vi "Process.vi"(8 "error in":errorcluster, 11 "instrument.Cryostation":refnum<class "instrument.Cryostation.lvclass">) -> (0 "error out":errorcluster, 3 "instrument.Cryostation out":refnum<class "instrument.Cryostation.lvclass">)   [LabVIEW 2019, in "instrument.Cryostation.lvclass"]
doc: "---------------------------------------------------------------\nJKI State Machine Objects™\nhttp://jki.net/state-machine-objects/\nCopyright (C) 2005-2015, JKI <info@jki.net>\nALL RIGHTS RESERVED"
uses:
  instrument.Cryostation.lvclass
  <vilib>/JKI/JKI SMO/SMO/SMO.lvclass
  C:/Program Files/National Instruments/LabVIEW 2019/user.lib/LevyLab/Instrument Framework/Instrument Types/Cryostat/Instrument.Cryostat.lvclass
  C:/Program Files/National Instruments/LabVIEW 2019/user.lib/LevyLab/Instrument Framework/Instrument/Instrument.lvclass
  C:/Program Files/National Instruments/LabVIEW 2019/vi.lib/JKI/JKI SMO/SMO/SMO.lvclass
  <userlib>/LevyLab/Debug/Debug.lvlib
  <userlib>/LevyLab/Instrument Framework/Instrument/Instrument.lvclass
  <userlib>/LevyLab/Instrument Framework/Instrument Types/Cryostat/Instrument.Cryostat.lvclass
panel:
  out "status string":string
  out "State History":string
  in  "STOP":bool
  # "Montana Cryostation"
  # "Montana Cryostation Monitor"
  # "THIS ONE IS NOT THE UI"
  # "For instructions on how to use the JKI State Machine Objects, examples and video tutorials, visit:\nhttp://jki.net/state-machine-objects/\n\nJKI State Machine Objects™\nhttp://jki.net/state-machine-objects/\nCopyright (C) 2005-2015, JKI <info@jki.net>\nALL RIGHTS RESERVED"
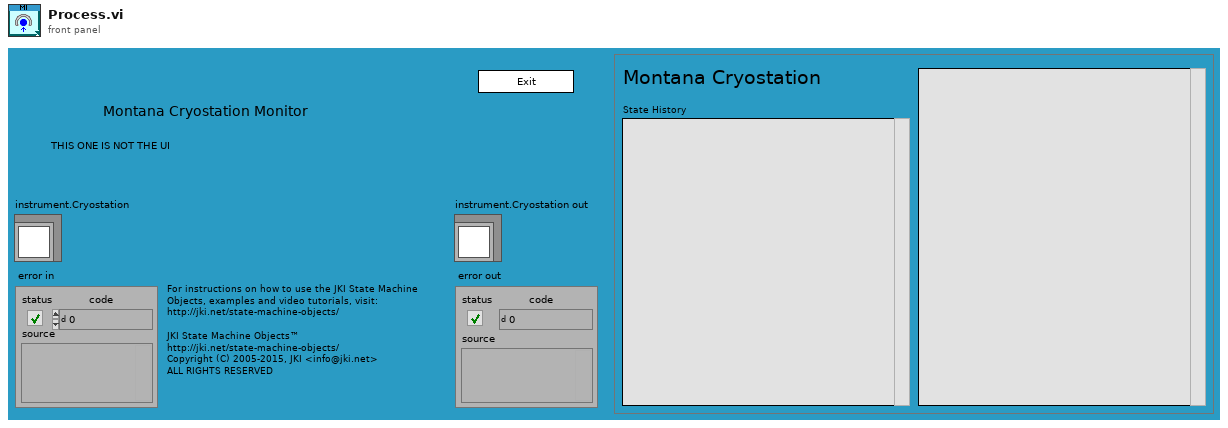
[diagram p1: front panel]
types:
  T1 = enum32{"invalid app kind", "Development System", "Run Time System", "Student Edition", "Embedded LabVIEW", "Evaluation", "Custom"}
  T2 = enum32{"Invalid", "Standard", "Closed", "Hidden", "Minimized", "Maximized"}
  T3 = cluster{"Core":cluster{"Current VI Reference":refnum<vi>, "Close Panel on Exit?":bool, "Shutdown?":bool, "Last Error":cluster{"error":errorcluster, "previous state":string, "remaining states":string}}, "SMO":refnum<class "instrument.Cryostation.lvclass">}
  T4 = cluster{"Current VI Reference":refnum<vi>, "Close Panel on Exit?":bool, "Shutdown?":bool, "Last Error":cluster{"error":errorcluster, "previous state":string, "remaining states":string}}
  T5 = typedef "Debug.lvlib/Attribute.Debug.lvclass/DebugBehavior.ctl" = enum16{"Normal", "Debug"}
  T6 = typedef "SMO.lvclass/Protected Events.ctl" = cluster{"StopProcesses":refnum<user-event>, "AbortProcesses":refnum<user-event>, "Config Changed":refnum<user-event>, "Dependency":refnum<user-event>}
  T7 = typedef "instrument.Cryostation.lvclass/Cryostation.getAll--cluster.ctl" = cluster{"Chamber Pressure (mTorr)":dbl, "Compressor Return Pressure (MPa)":dbl, "Compressor Supply Pressure (MPa)":dbl, "Compressor Speed (Hz)":dbl, "Cold Head Speed (Hz)":dbl, "Platform Heater Power (W)":dbl, "Platform Stability (K)":dbl, "Platform Temperature (K)":dbl, "Stage 1 Heater Power (W)":dbl, "Stage 1 Temperature (K)":dbl, "Stage 2 Heater Power (W)":dbl, "Stage 2 Temperature (K)":dbl, "Sample Stability (K)":dbl, "Sample Temperature (K)":dbl, "Temperature Set Point (K)":dbl, "User Stability (K)":dbl, "User Temperature (K)":dbl, "User Temperature Set Point (K)":dbl, "Alarm State":string, "Compressor Run State":string, "Case Valve State":string, "Idle State":string, "Nitrogen State":string, "Vent Valve State":string}
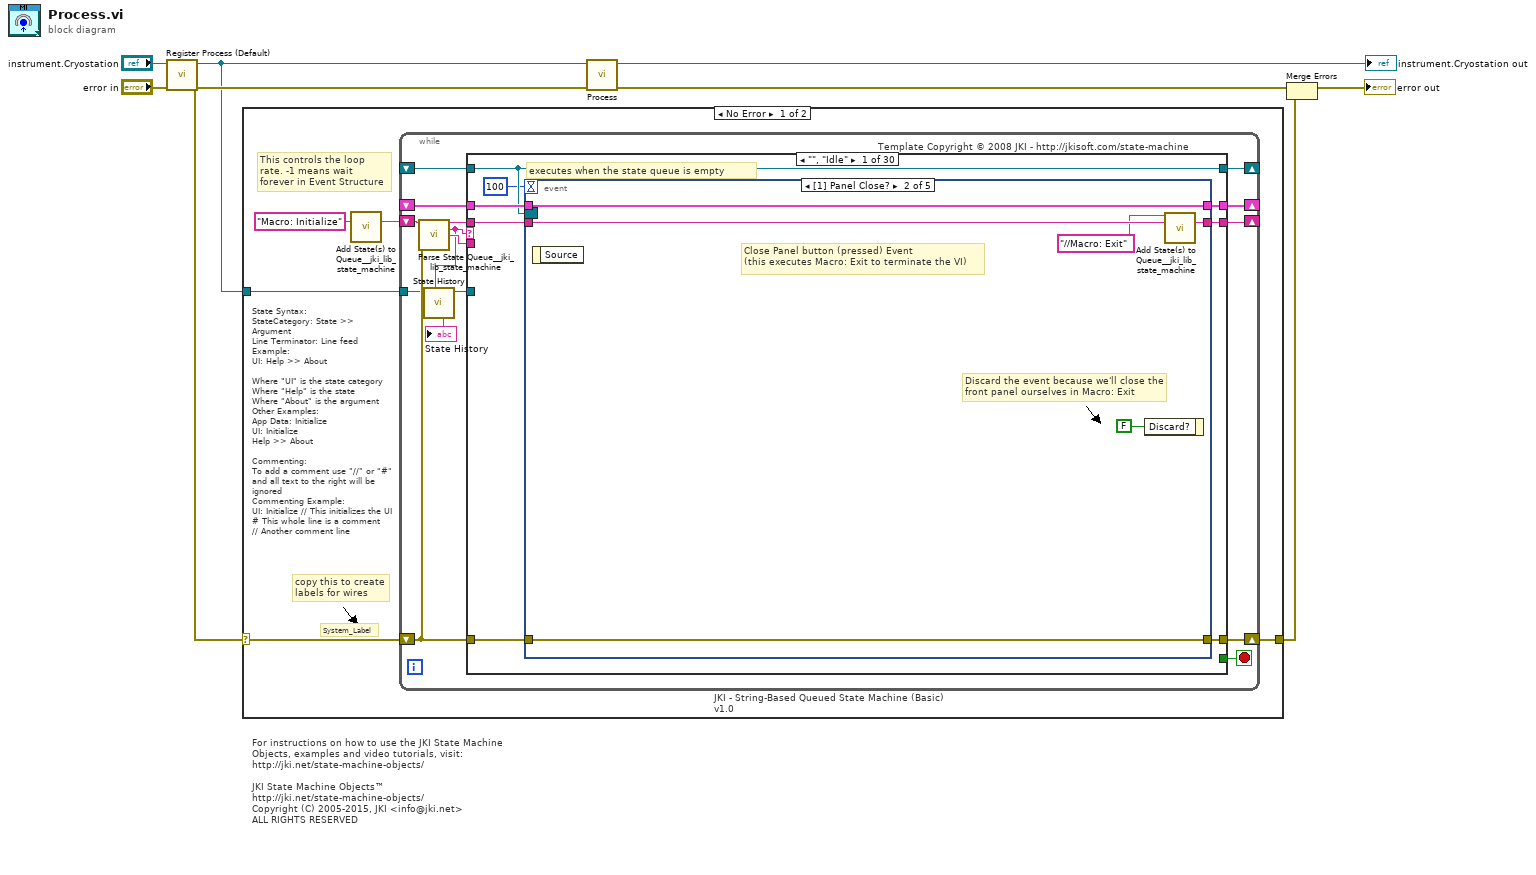
[diagram p0: block diagram]
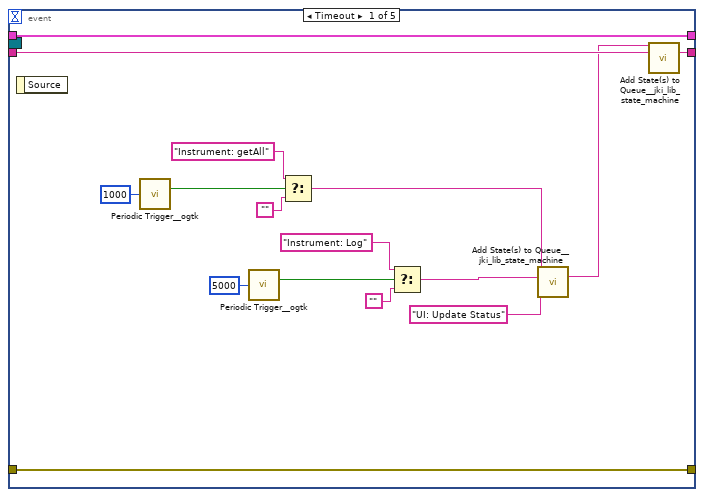
[diagram p2: hidden frame]
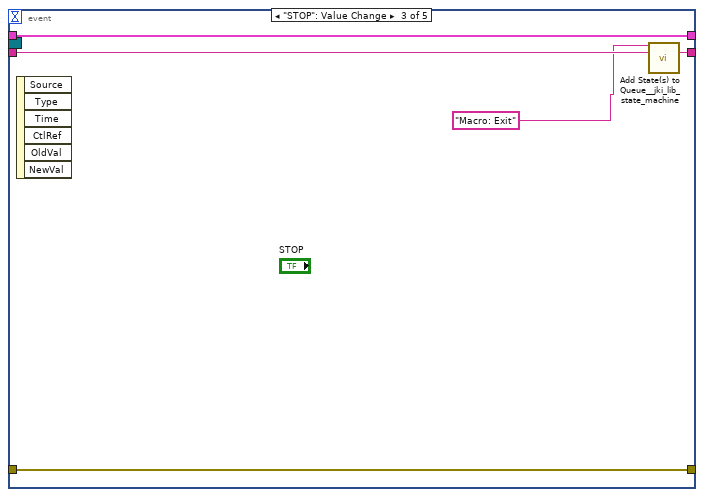
[diagram p3: hidden frame]
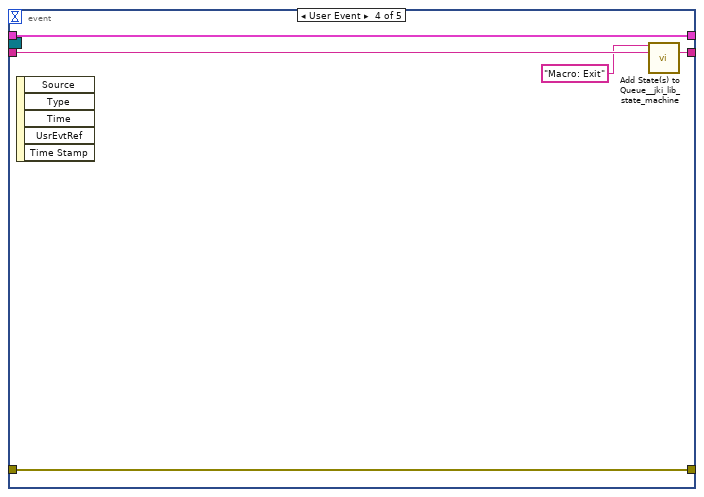
[diagram p4: hidden frame]
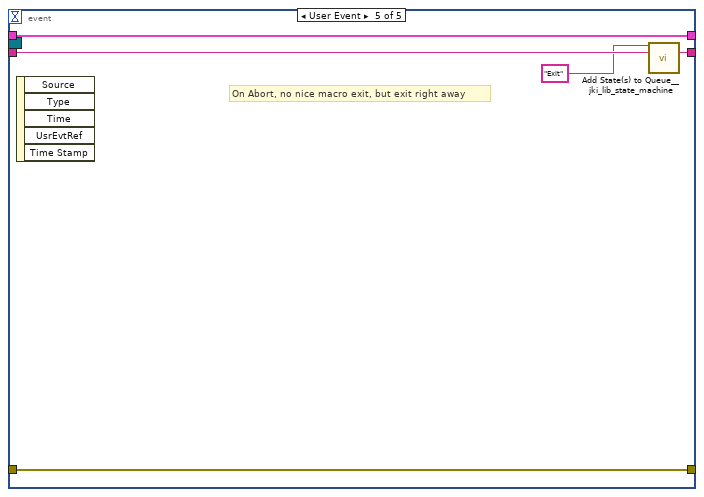
[diagram p5: hidden frame]
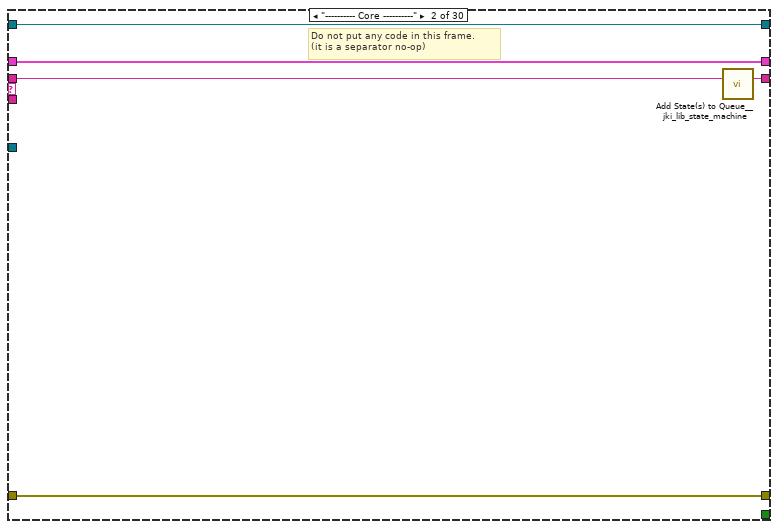
[diagram p6: hidden frame]
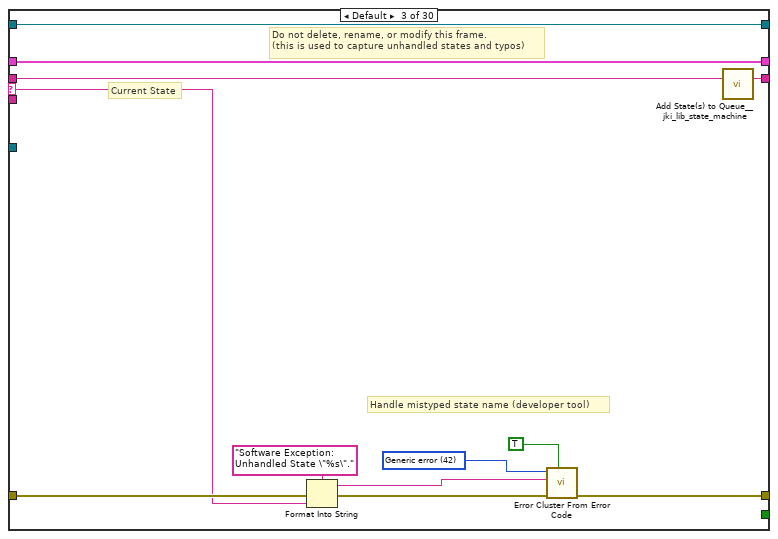
[diagram p7: hidden frame]
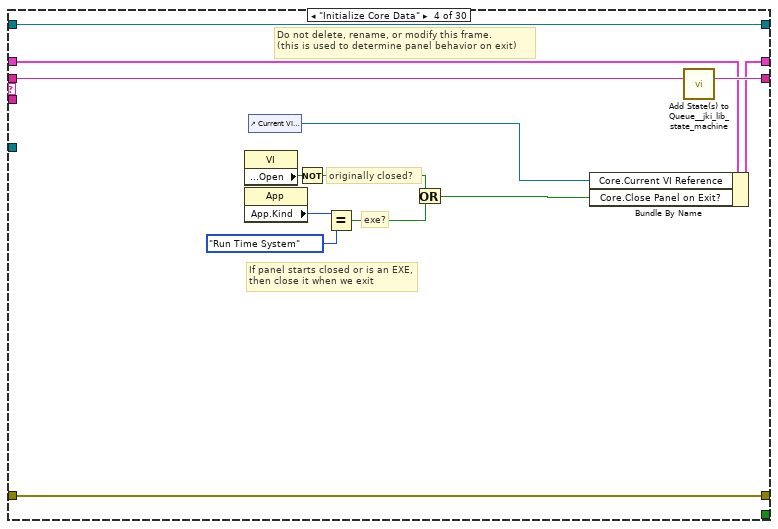
[diagram p8: hidden frame]
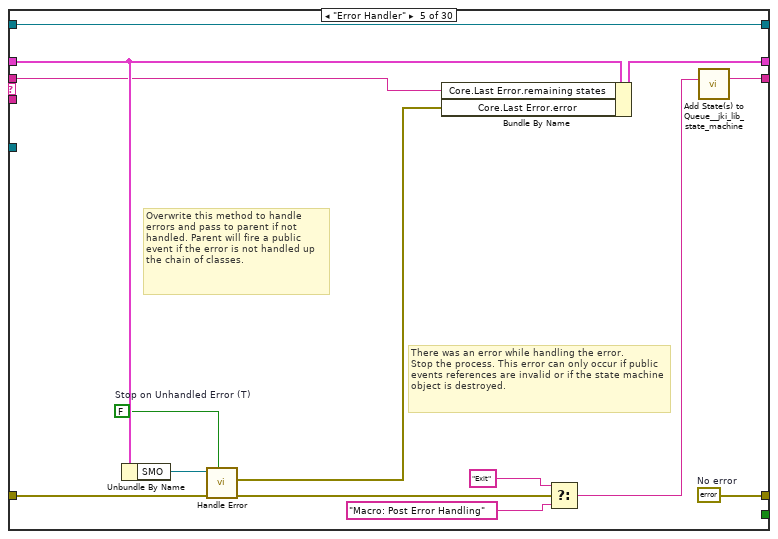
[diagram p9: hidden frame]
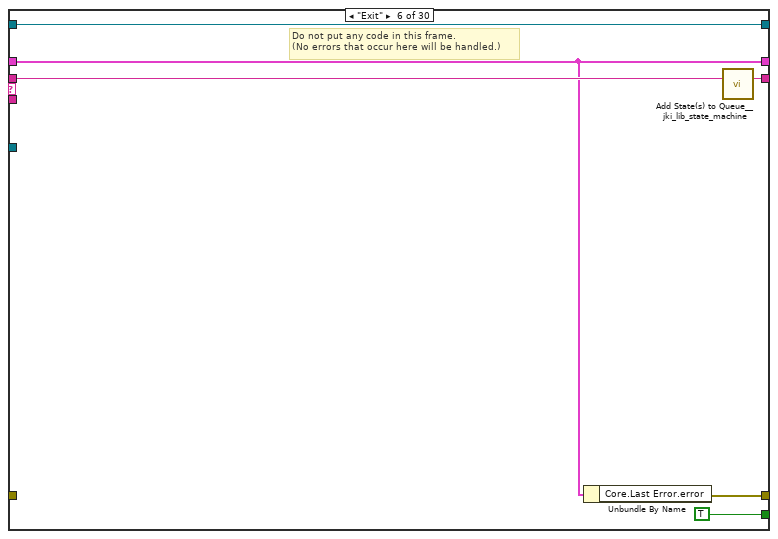
[diagram p10: hidden frame]
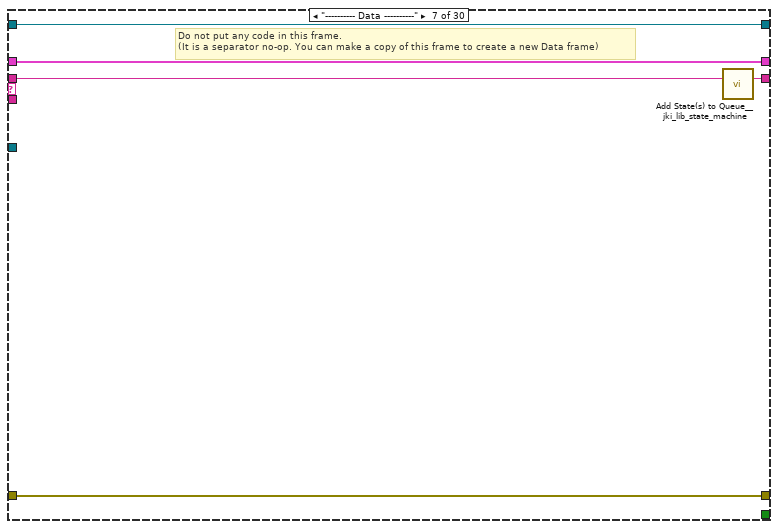
[diagram p11: hidden frame]
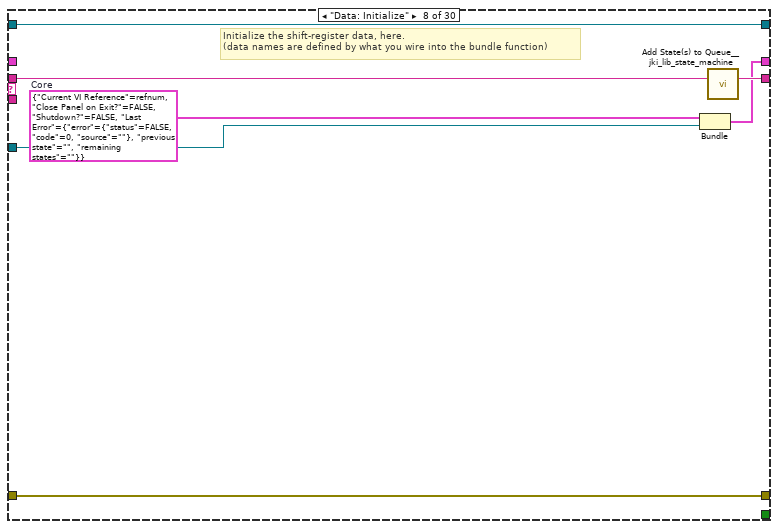
[diagram p12: hidden frame]
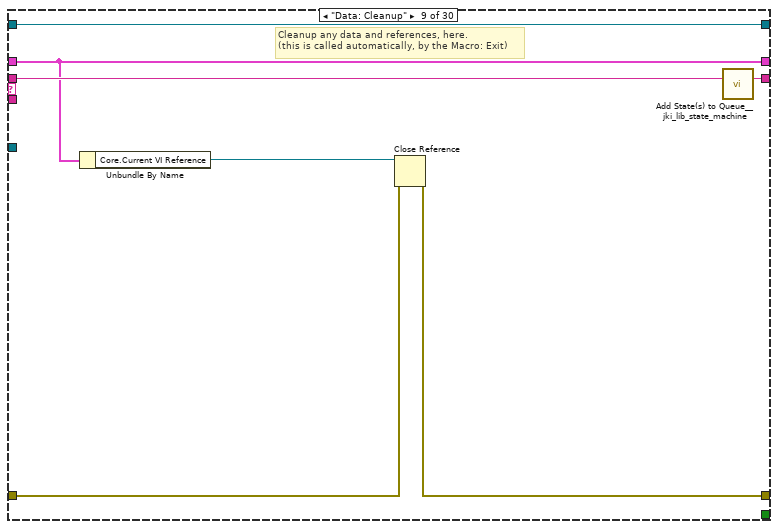
[diagram p13: hidden frame]
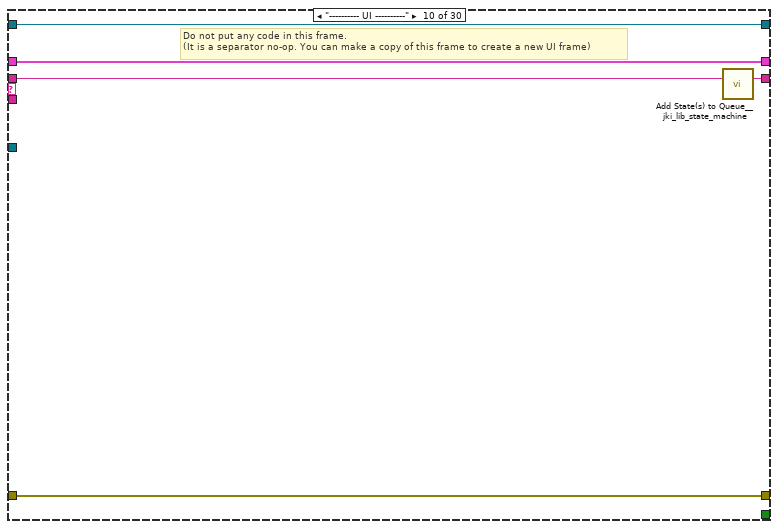
[diagram p14: hidden frame]
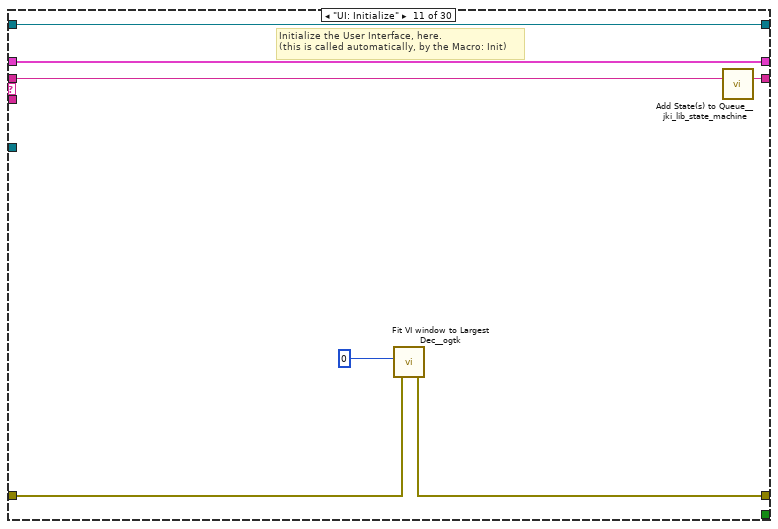
[diagram p15: hidden frame]
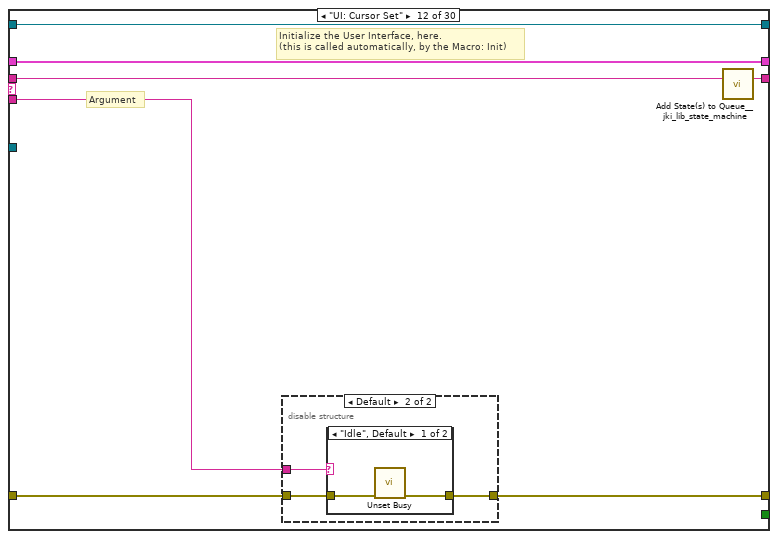
[diagram p16: hidden frame]
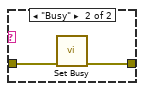
[diagram p18: hidden frame]
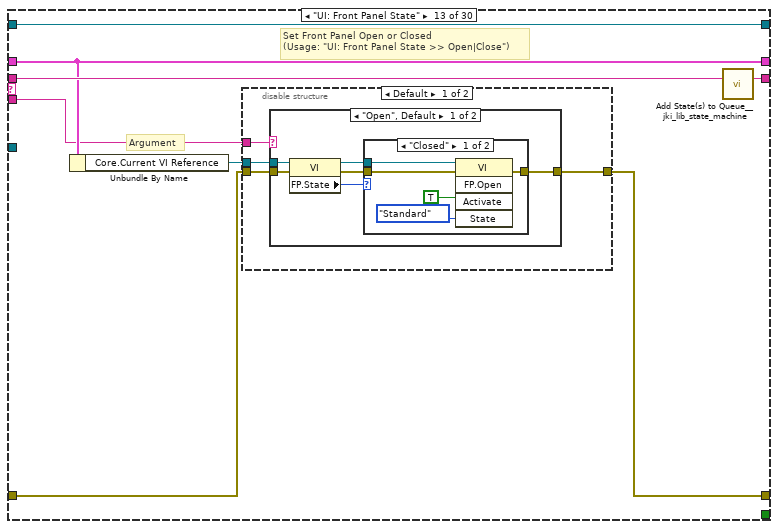
[diagram p19: hidden frame]
diagram:
  # "For instructions on how to use the JKI State Machine Objects, examples and video tutorials, visit:\nhttp://jki.net/state-machine-objects/\n\nJKI State Machine Objects™\nhttp://jki.net/state-machine-objects/\nCopyright (C) 2005-2015, JKI <info@jki.net>\nALL RIGHTS RESERVED"
  n1 = call <vilib>:"Register Process (Default).vi"("error in (no error)"="error in", "SMO"="instrument.Cryostation") -> ("error out"=w5:errorcluster, "SelfRef"=w4:refnum<class "instrument.Cryostation.lvclass">)  [unwired: 8 in]
  n2 = case shown="No Error" w5 {
    selector: w5 -> [w10 w373]
    tunnel: w4 -> [w11 _]
    tunnel: [w9 w373] -> w1
    frame No Error {
      # "State Syntax:\nStateCategory: State >> Argument\nLine Terminator: Line feed\nExample:\nUI: Help >> About\n\nWhere \"UI\" is the state category\nWhere \"Help\" is the state\nWhere \"About\" is the argument\nOther Examples:\nApp Data: Initialize\nUI: Initialize\nHelp >> About\n\nCommenting:\nTo add a comment use \"//\" or \"#\" and all text to the right will be ignored\nCommenting Example:\nUI: Initialize // This initializes the UI\n# This whole line is a comment\n// Another comment line"
      # "copy this to create labels for wires"
      # "This controls the loop rate. -1 means wait forever in Event Structure"
      # "System_Label"
      n3 = call <vilib>:"Add State(s) to Queue__jki_lib_state_machine.vi"("State(s) in (\"\")"="Macro: Initialize") -> ("States Out"=w13:string)  [unwired: 14 in]
      n4 = while "JKI - String-Based Queued State Machine (Basic) v1.0" {
        shift-right: [w22] -> _
        shift-left: _ -> [w18]
        shift-right: [w25] -> w9
        shift-left: w10 -> [w21]
        shift-right: [w24] -> _
        shift-left: w13 -> [w26]
        tunnel: w11 -> [w14]
        shift-right: [w20] -> _
        shift-left: _ -> [w19]
        stop <- w23 stop-if-true
        # "Template Copyright © 2008 JKI - http://jkisoft.com/state-machine"
        n5 = call <vilib>:"Parse State Queue__jki_lib_state_machine.vi"("State Queue"=w26, "Error In (no error)"=w21) -> ("Remaining States"=w28:string, "Current State"=w17:string, "Arguments"=w27:string)  [unwired: 11 in]
        n6 = call <userlib>:"State History.vi"("Current State"=w17, "SMO"=w14) -> ("SMO"=w15:refnum<class "instrument.Cryostation.lvclass">, "History"=→"State History":string)  [unwired: 8 in]
        n7 = case shown="\"\", \"Idle\"" w17 {
          selector: w17 -> [_ _ w80 _ _ _ _ _ _ _ _ _ _ _ _ _ _ _ _ _ _ _ _ _ _ _ _ _ _ _]
          tunnel: w28 -> [w36 w78 w84 w103 w105 w123 w128 w135 w142 w147 w154 w161 w177 w212 w221 w226 w235 w238 w257 w287 w292 w303 w308 w318 w324 w329 w338 w350 w363 w372]
          tunnel: w27 -> [_ _ _ _ _ _ _ _ _ _ _ w155 w171 _ w213 _ _ _ _ _ _ _ _ _ _ _ _ _ _ _]
          tunnel: w18 -> [w34 w75 w82 w94 w112 w119 w125 _ w138 w144 w152 w159 w173 w209 w218 w223 w231 w239 w253 w272 w289 w300 w305 w316 w322 w326 w332 w345 w359 w366]
          tunnel: [w33 w76 w86 w100 w113 w118 w126 w129 w139 w145 w149 w156 w174 w207 w219 w224 w233 w246 w255 w285 w290 w294 w306 w311 w320 w327 w331 w339 w352 w365] -> w25
          tunnel: w21 -> [w32 w76 w85 w100 w114 _ w126 w129 w136 w145 w148 w157 w175 w205 w219 w224 w233 w246 w256 w285 w290 w295 w306 w312 w320 w327 w330 w344 w354 w364]
          tunnel: [w35 w77 w83 w102 w117 w122 w127 w134 w141 w146 w153 w160 w176 w211 w220 w225 w234 w247 w266 w286 w291 w302 w307 w317 w323 w328 w337 w349 w362 w371] -> w24
          tunnel: [_ _ _ _ _ TRUE _ _ _ _ _ _ _ _ _ _ _ _ _ _ _ _ _ _ _ _ _ _ _ _] -> w23
          tunnel: [w31 w75 w82 w101 w111 w119 w125 w131 w138 w144 w152 w159 w173 w209 w218 w223 w231 w237 w254 w273 w289 w300 w305 w316 w322 w326 w333 w346 w360 w367] -> w22
          tunnel: w15 -> [_ _ _ _ _ _ _ w130 _ _ _ _ _ _ _ _ _ _ _ _ _ _ _ _ _ _ _ _ _ _]
          tunnel: [w30 w74 w79 w91 w116 w120 w124 w133 w137 w143 w151 w158 w170 w210 w217 w222 w232 w245 w265 w279 w288 w301 w304 w315 w321 w325 w336 w348 w361 w370] -> w20
          tunnel: w19 -> [w30 w74 w79 w91 w116 w120 w124 w133 w137 w143 w151 w158 w170 w210 w217 w222 w232 w245 w265 w279 w288 w301 w304 _ w321 w325 w336 w348 w361 w370]
          frame "", "Idle" {
            # "executes when the state queue is empty"
            n8 = event shown="[1] Panel Close?" {
              selector: w30 -> [_ _ _ _ _]
              dyn-events: _ -> [_ _ _ _ _]
              timeout: 100 -> [_ _ _ _ _]
              tunnel: w36 -> [w52 w58 w63 w68 w73]
              tunnel: [w51 w57 w62 w67 w72] -> w35
              tunnel: w34 -> [w50 w55 w60 w65 w70]
              tunnel: [w49 w56 w61 w66 w71] -> w33
              tunnel: w32 -> [w49 w56 w61 w66 w71]
              tunnel: [w50 w55 w60 w65 w70] -> w31
              event Timeout {
                n9 = event-data() -> ()  [unwired: 1 in, 1 out]
                n10 = call <userlib>:"Periodic Trigger__ogtk.vi"("time (ms)"=u32 1000) -> ("Triggered"=w48:bool)  [unwired: 12 in, 2 out]
                n11 = call <userlib>:"Periodic Trigger__ogtk.vi"("time (ms)"=u32 5000) -> ("Triggered"=w40:bool)  [unwired: 12 in, 2 out]
                n12 = Select(t="Instrument: getAll", s=w48, f="") -> (s? t:f=w43:string)
                n13 = Select(t="Instrument: Log", s=w40, f="") -> (s? t:f=w38:string)
                n14 = call <vilib>:"Add State(s) to Queue__jki_lib_state_machine.vi"("State(s) in Front (\"\")"=w43, "State(s) in (\"\")"=w38, "State(s) at Back (\"\")"="UI: Update Status") -> ("States Out"=w37:string)  [unwired: 12 in]
                n15 = call <vilib>:"Add State(s) to Queue__jki_lib_state_machine.vi"("State(s) in Front (\"\")"=w37, "State(s) in (\"\")"=w52) -> ("States Out"=w51:string)  [unwired: 13 in]
              }
              event Panel Close? {
                # "Discard the event because we'll close the front panel ourselves in Macro: Exit"
                # "Close Panel button (pressed) Event\n(this executes Macro: Exit to terminate the VI)"
                n16 = event-data() -> ()  [unwired: 1 in, 1 out]
                n17 = event-data("Discard?"=FALSE) -> ()  [unwired: 1 in, 1 out]
                n18 = call <vilib>:"Add State(s) to Queue__jki_lib_state_machine.vi"("State(s) in Front (\"\")"="//Macro: Exit", "State(s) in (\"\")"=w58) -> ("States Out"=w57:string)  [unwired: 13 in]
              }
              event "STOP": Value Change {
                n19 = event-data() -> ()  [unwired: 1 in, 6 out]
                n20 = call <vilib>:"Add State(s) to Queue__jki_lib_state_machine.vi"("State(s) in Front (\"\")"="Macro: Exit", "State(s) in (\"\")"=w63) -> ("States Out"=w62:string)  [unwired: 13 in]
              }
              event User Event {
                n21 = event-data() -> ()  [unwired: 1 in, 5 out]
                n22 = call <vilib>:"Add State(s) to Queue__jki_lib_state_machine.vi"("State(s) in Front (\"\")"="Macro: Exit", "State(s) in (\"\")"=w68) -> ("States Out"=w67:string)  [unwired: 13 in]
              }
              event User Event {
                # "On Abort, no nice macro exit, but exit right away"
                n23 = event-data() -> ()  [unwired: 1 in, 5 out]
                n24 = call <vilib>:"Add State(s) to Queue__jki_lib_state_machine.vi"("State(s) in Front (\"\")"="Exit", "State(s) in (\"\")"=w73) -> ("States Out"=w72:string)  [unwired: 13 in]
              }
            }
          }
          frame "---------- Core ----------" {
            # "Do not put any code in this frame.\n(it is a separator no-op)"
            n25 = call <vilib>:"Add State(s) to Queue__jki_lib_state_machine.vi"("State(s) in (\"\")"=w78) -> ("States Out"=w77:string)  [unwired: 14 in]
          }
          frame Default {
            w89 = 42 items=["No error", "Argument error", "Memory is full", "Out of zone", "End of file", "File already open", "Generic file I/O error", "File not found", "File permission error", "Disk is full", "Duplicate path", "Too many files open", "System feature not enabled", "Resource file not found", "Cannot add resource", "Resource not found", "Image not found", "Image memory error", "Pen does not exist", "Config type invalid", "Config token not found", "Config parse error", "Config memory error", "Bad external code format", "Bad external code offset", "External code not present", "Null window", "Destroy window error", "Null menu", "Print aborted", "Bad print record", "Print driver error", "Windows error during printing", "Memory error during printing", "Print dialog error", "Generic print error", "Invalid device refnum", "Device not found", "Device parameter error", "Device unit error", "Cannot open device", "Device call aborted", "Generic error", "Cancelled by user", "Object ID too low", "Object ID too high", "Object not in heap", "Unknown heap", "Unknown object (invalid DefProc)", "Unknown object (DefProc not in table)", "Message out of range", "Invalid (null) method", "Unknown message", "Manager call not supported", "Bad address", "Network operation in progress", "Network operation timed out", "Connection is busy", "Network attribute not supported", "Network error", "Address in use", "System out of memory", "Connection aborted", "Connection refused", "Not connected", "Already connected", "Connection closed", "Initialization error (interapplication manager)", "Bad occurrence", "Wait on unbound occurrence handler", "Occurrence queue overflow", "Datalog type conflict", "Unused", "Unrecognized type (interapplication manager)", "Memory corrupt", "Failed to make temporary DLL", "Old CIN version", "Drag socket not found", "Failed to load drop-object", "Failed to register OLE object", "Failed to release OLE object", "Format specifier type mismatch", "Unknown format specifier", "Too few format specifiers", "Too many format specifiers", "Scan failed", "Newer CIN version", "Error converting to variant", "Runtime menu error", "Password tampered", "Variant attribute not found", "Incompatible variant data type", "Event data is not available", "Event Store is not present", "Occurrence is not found", "Event Queue is not created", "Event info is not available", "Refnum passed is NULL", "Error retrieving Class GUID", "Error retrieving CoClass GUID", "Error retrieving TypeLib GUID.", "Bad built application magic bytes.", "Specific driver is different from the specific driver associated with the Logical Name.", "There is no session opened to the class driver.", "Max Error", "MAX - Error with config objects", "MAX - Error loading configuration", "MAX - Group not supported"]
            # "Current State"
            # "Do not delete, rename, or modify this frame.\n(this is used to capture unhandled states and typos)"
            # "Handle mistyped state name (developer tool)"
            n26 = Format Into String(format string="Software Exception: Unhandled State \"%s\"." ("message"), error in=w85, w80) -> (resulting string=w88:string, error out=w87:errorcluster)  [unwired: 1 in]
            n27 = call <vilib>:"Error Cluster From Error Code.vi"("show call chain? (False)"=TRUE, "error in (no error)"=w87, "error message (\"\")"=w88, "error code (0)"=w89) -> ("error out"=w86:errorcluster)  [unwired: 5 in]
            n28 = call <vilib>:"Add State(s) to Queue__jki_lib_state_machine.vi"("State(s) in (\"\")"=w84) -> ("States Out"=w83:string)  [unwired: 14 in]
          }
          frame "Initialize Core Data" {
            # "Do not delete, rename, or modify this frame.\n(this is used to determine panel behavior on exit)"
            # "originally closed?"
            # "exe?"
            # "If panel starts closed or is an EXE, then close it when we exit"
            n29 = property class="VI"() -> ("Front Panel.Open"=w99:bool)  [unwired: 2 in, 2 out]
            n30 = property class="App"() -> ("App.Kind"=w98:T1)  [unwired: 2 in, 2 out]
            n31 = control-ref of="Current VI Reference"() -> (w92:refnum<vi>)
            n32 = Not(x=w99) -> (.not. x?=w96:bool)
            n33 = Equal?(x=w98, y=T1."Run Time System" ("Application:Kind")) -> (x = y?=w95:bool)
            n34 = Or(x=w96, y=w95) -> (x .or. y?=w93:bool)
            n35 = Bundle By Name(cluster=w94, "Core.Current VI Reference"=w92, "Core.Close Panel on Exit?"=w93) -> (w101:T3)
            n36 = call <vilib>:"Add State(s) to Queue__jki_lib_state_machine.vi"("State(s) in (\"\")"=w103) -> ("States Out"=w102:string)  [unwired: 14 in]
          }
          frame "Error Handler" {
            w108 = FALSE  # Stop on Unhandled Error (T)
            w113 = errorcluster {"status"=FALSE, "code"=0, "source"=""}  # No error
            # "There was an error while handling the error.\nStop the process. This error can only occur if public events references are invalid or if the state machine object is destroyed."
            # "Overwrite this method to handle errors and pass to parent if not handled. Parent will fire a public event if the error is not handled up the chain of classes."
            n37 = Unbundle By Name(w112) -> ("SMO"=w115:refnum<class "instrument.Cryostation.lvclass">)
            n38 = call-dynamic "Handle Error.vi"("Stop on Unhandled Error (T)"=w108, "error in"=w114, "SMO"=w115) -> ("handling error"=w109:errorcluster, "Unhandled error"=w107:errorcluster)  [unwired: 6 in, 1 out]
            n39 = Bundle By Name(cluster=w112, "Core.Last Error.remaining states"=w105, "Core.Last Error.error"=w107) -> (w111:T3)
            n40 = Select(t="Exit", s=w109, f="Macro: Post Error Handling") -> (s? t:f=w104:string)
            n41 = call <vilib>:"Add State(s) to Queue__jki_lib_state_machine.vi"("State(s) in (\"\")"=w104) -> ("States Out"=w117:string)  [unwired: 14 in]
          }
          frame "Exit" {
            # "Do not put any code in this frame.\n(No errors that occur here will be handled.)"
            n42 = Unbundle By Name(w119) -> ("Core.Last Error.error"=w118:errorcluster)
            n43 = call <vilib>:"Add State(s) to Queue__jki_lib_state_machine.vi"("State(s) in (\"\")"=w123) -> ("States Out"=w122:string)  [unwired: 14 in]
          }
          frame "---------- Data ----------" {
            # "Do not put any code in this frame.\n(It is a separator no-op. You can make a copy of this frame to create a new Data frame)"
            n44 = call <vilib>:"Add State(s) to Queue__jki_lib_state_machine.vi"("State(s) in (\"\")"=w128) -> ("States Out"=w127:string)  [unwired: 14 in]
          }
          frame "Data: Initialize" {
            w132 = T4 {"Current VI Reference"=refnum, "Close Panel on Exit?"=FALSE, "Shutdown?"=FALSE, "Last Error"={"error"={"status"=FALSE, "code"=0, "source"=""}, "previous state"="", "remaining states"=""}}  # Core
            # "Initialize the shift-register data, here.\n(data names are defined by what you wire into the bundle function)"
            n45 = Bundle("Core"=w132, "SMO"=w130) -> (w131:T3)  [unwired: 1 in]
            n46 = call <vilib>:"Add State(s) to Queue__jki_lib_state_machine.vi"("State(s) in (\"\")"=w135) -> ("States Out"=w134:string)  [unwired: 14 in]
          }
          frame "Data: Cleanup" {
            # "Cleanup any data and references, here.\n(this is called automatically, by the Macro: Exit)"
            n47 = Unbundle By Name(w138) -> ("Core.Current VI Reference"=w140:refnum<vi>)
            n48 = Close Reference(reference=w140, error in (no error)=w136) -> (error out=w139:errorcluster)
            n49 = call <vilib>:"Add State(s) to Queue__jki_lib_state_machine.vi"("State(s) in (\"\")"=w142) -> ("States Out"=w141:string)  [unwired: 14 in]
          }
          frame "---------- UI ----------" {
            # "Do not put any code in this frame.\n(It is a separator no-op. You can make a copy of this frame to create a new UI frame)"
            n50 = call <vilib>:"Add State(s) to Queue__jki_lib_state_machine.vi"("State(s) in (\"\")"=w147) -> ("States Out"=w146:string)  [unwired: 14 in]
          }
          frame "UI: Initialize" {
            # "Initialize the User Interface, here.\n(this is called automatically, by the Macro: Init)"
            n51 = call <userlib>:"Fit VI window to Largest Dec__ogtk.vi"("error in (no error)"=w148, "border spacing (2 px)"=0) -> ("error out"=w149:errorcluster)  [unwired: 4 in, 1 out]
            n52 = call <vilib>:"Add State(s) to Queue__jki_lib_state_machine.vi"("State(s) in (\"\")"=w154) -> ("States Out"=w153:string)  [unwired: 14 in]
          }
          frame "UI: Cursor Set" {
            # "Argument"
            # "Initialize the User Interface, here.\n(this is called automatically, by the Macro: Init)"
            n53 = disable-structure shown="Default" {
              disable-tunnel: w157 -> [w162 w165]
              disable-tunnel: [w162 w164] -> w156
              disable-tunnel: w155 -> [_ w163]
              frame condition #0 {
              }
              frame condition #1 (active) {
                n54 = case shown="\"Idle\", Default" w163 {
                  tunnel: w165 -> [w167 w169]
                  tunnel: [w166 w168] -> w164
                  frame "Idle", Default {
                    n55 = call <vilib>:"Unset Busy.vi"("error in (no error)"=w167) -> ("error out"=w166:errorcluster)  [unwired: 10 in]
                  }
                  frame "Busy" {
                    n56 = call <vilib>:"Set Busy.vi"("error in (no error)"=w169) -> ("error out"=w168:errorcluster)  [unwired: 9 in, 1 out]
                  }
                }
              }
            }
            n57 = call <vilib>:"Add State(s) to Queue__jki_lib_state_machine.vi"("State(s) in (\"\")"=w161) -> ("States Out"=w160:string)  [unwired: 14 in]
          }
          frame "UI: Front Panel State" {
            # "Argument"
            # "Set Front Panel Open or Closed\n(Usage: \"UI: Front Panel State >> Open|Close\")"
            n58 = Unbundle By Name(w173) -> ("Core.Current VI Reference"=w172:refnum<vi>)
            n59 = disable-structure shown="Default" {
              disable-tunnel: w175 -> [w181 w204]
              disable-tunnel: [w180 w204] -> w174
              disable-tunnel: w172 -> [w179 _]
              disable-tunnel: w171 -> [w178 _]
              frame condition #0 (active) {
                n60 = case shown="\"Open\", Default" w178 {
                  tunnel: w181 -> [w185 w198]
                  tunnel: [w187 w199] -> w180
                  tunnel: w179 -> [w186 w196]
                  frame "Open", Default {
                    n61 = property class="VI"(reference=w186, error in=w185) -> (reference out=w183:refnum<vi>, error out=w184:errorcluster, "FP.State"=w182:T2)
                    n62 = case shown="\"Closed\"" w182 {
                      tunnel: [w190 w193] -> w187
                      tunnel: w184 -> [w189 w193]
                      tunnel: w183 -> [w188 _]
                      frame "Closed" {
                        n63 = invoke class="VI" method="FP.Open"(reference=w188, error in=w189, "Activate"=TRUE, "State"=T2."Standard") -> (error out=w190:errorcluster)  [unwired: 1 in, 4 out]
                      }
                      frame Default {
                      }
                    }
                  }
                  frame "Close" {
                    n64 = property class="VI"(reference=w196, error in=w198) -> (reference out=w195:refnum<vi>, error out=w197:errorcluster, "FP.State"=w194:T2)
                    n65 = case shown="\"Invalid\", \"Closed\"" w194 {
                      tunnel: [w200 w203] -> w199
                      tunnel: w197 -> [w200 w202]
                      tunnel: w195 -> [_ w201]
                      frame "Invalid", "Closed" {
                      }
                      frame Default {
                        n66 = invoke class="VI" method="FP.Close"(reference=w201, error in=w202) -> (error out=w203:errorcluster)  [unwired: 1 in, 2 out]
                      }
                    }
                  }
                }
              }
              frame condition #1 {
              }
            }
            n67 = call <vilib>:"Add State(s) to Queue__jki_lib_state_machine.vi"("State(s) in (\"\")"=w177) -> ("States Out"=w176:string)  [unwired: 14 in]
          }
          frame "UI: Update Status" {
            n68 = Unbundle By Name(w209) -> ("SMO"=w208:refnum<class "instrument.Cryostation.lvclass">)
            n69 = call "Cryostation.GetAlltoStatusString.vi"("error in (no error)"=w205, "instrument.Cryostation in"=w208) -> ("error out"=w207:errorcluster, "status string"=→"status string":string)  [unwired: 7 in, 1 out]
            n70 = call <vilib>:"Add State(s) to Queue__jki_lib_state_machine.vi"("State(s) in (\"\")"=w212) -> ("States Out"=w211:string)  [unwired: 14 in]
          }
          frame "UI: Wait" {
            n71 = Scan From String(format string="%d", input string=w213, default 1=u32 0 ("default value 1")) -> (output 1=w214:u32)  [unwired: 2 in, 3 out]
            n72 = Wait (ms)(milliseconds to wait=w214) -> ()  [unwired: 1 out]
            n73 = call <vilib>:"Add State(s) to Queue__jki_lib_state_machine.vi"("State(s) in (\"\")"=w221) -> ("States Out"=w220:string)  [unwired: 14 in]
          }
          frame "---------- Macro ----------" {
            # "Do not put any code in this frame.\n(It is a separator no-op. You can make a copy of this frame to create a new Macro frame)"
            n74 = call <vilib>:"Add State(s) to Queue__jki_lib_state_machine.vi"("State(s) in (\"\")"=w226) -> ("States Out"=w225:string)  [unwired: 14 in]
          }
          frame "Macro: Initialize" {
            # "Initialization Macro\n(This is called once, when the VI starts)"
            n75 = call <vilib>:"Add State(s) to Queue__jki_lib_state_machine.vi"("State(s) in Front (\"\")"="Data: Initialize\nInitialize Core Data\nEvents: Register", "State(s) in (\"\")"="Process: Sync", "State(s) at Back (\"\")"="UI: Initialize\nUI: Front Panel State >> Close\nMacro: Debug\nInstrument: Open\nInstrument: getAll") -> ("States Out"=w228:string)  [unwired: 12 in]
            n76 = call <vilib>:"Add State(s) to Queue__jki_lib_state_machine.vi"("State(s) in Front (\"\")"=w228, "State(s) in (\"\")"=w235) -> ("States Out"=w234:string)  [unwired: 13 in]
          }
          frame "Macro: Post Error Handling" {
            # "Clear Last Error?"
            n77 = Unbundle By Name(w239) -> ("Core.Last Error.remaining states"=w243:string, "Core.Shutdown?"=w244:bool)
            n78 = Unbundle By Name(w239) -> ("Core.Last Error.error"=w241:errorcluster)
            n79 = case shown="False" FALSE {
              tunnel: w241 -> [w248 _]
              tunnel: [w248 _] -> w240
              frame False {
              }
              frame True {
              }
            }
            n80 = case shown="True" w244 {
              tunnel: w243 -> [w249 w251]
              tunnel: [w249 w250] -> w236
              frame False {
                # "These are the remaining states (at the moment the error occured). States can be altered according to business logic."
                # "NOT SHUTTING DOWN"
              }
              frame True {
                # "Developer can decide to alter the states but should be aware that during the shutdown process, there are certain states that must be run for the SMO to properly shut itself (and this process) down. As such, one can add states to perform additional clean-ups, but should append the remaining state to be executed."
                # "SHUTTING DOWN"
                n81 = call <vilib>:"Add State(s) to Queue__jki_lib_state_machine.vi"("State(s) in (\"\")"=w251) -> ("States Out"=w250:string)  [unwired: 14 in]
              }
            }
            n82 = Bundle By Name(cluster=w239, "Core.Last Error.error"=w240) -> (w237:T3)
            n83 = call <vilib>:"Add State(s) to Queue__jki_lib_state_machine.vi"("State(s) in Front (\"\")"=w236, "State(s) in (\"\")"=w238) -> ("States Out"=w247:string)  [unwired: 13 in]
          }
          frame "Macro: Debug" {
            # "exe?"
            # "If pane is an EXE, then close it when we exit"
            # "Macro: Debug\n(get debug behavior, determine UI and determine shutdown behavior)"
            n84 = Unbundle By Name(w253) -> ("Core.Close Panel on Exit?"=w259:bool, "SMO"=w264:refnum<class "instrument.Cryostation.lvclass">)
            n85 = property class="App"() -> ("App.Kind"=w262:T1)  [unwired: 2 in, 2 out]
            n86 = Equal?(x=w262, y=T1."Run Time System" ("Application:Kind")) -> (x = y?=w258:bool)
            n87 = call <userlib>:"Get Debug Mode.vi"("error in (no error)"=w256, "SMO"=w264) -> ("error out"=w255:errorcluster, "Behavior"=w263:T5)  [unwired: 7 in, 1 out]
            n88 = case shown="\"Debug\"" w263 {
              tunnel: [w267 w269] -> w260
              tunnel: w259 -> [w267 _]
              tunnel: w258 -> [_ w271]
              tunnel: [_ "UI: Front Panel State >> Open\nUI: Wait >> 1000"] -> w252
              frame "Normal", Default {
                # "respect core.close"
              }
              frame "Debug" {
                # "keep panel open\nunless exe"
                n89 = Or(x=w271, y=FALSE) -> (x .or. y?=w269:bool)
              }
            }
            n90 = Bundle By Name(cluster=w253, "Core.Close Panel on Exit?"=w260) -> (w254:T3)
            n91 = call <vilib>:"Add State(s) to Queue__jki_lib_state_machine.vi"("State(s) in Front (\"\")"=w252, "State(s) in (\"\")"=w257) -> ("States Out"=w266:string)  [unwired: 13 in]
          }
          frame "Macro: Exit" {
            # "Exit Macro\n(This is called once, when the VI exits)"
            n92 = Unbundle By Name(w272) -> ("Core.Close Panel on Exit?"=w284:bool)
            n93 = Bundle By Name(cluster=w272, "Core.Shutdown?"=TRUE) -> (w273:T3)
            n94 = Select(t="UI: Front Panel State >> Close", s=w284, f="") -> (s? t:f=w281:string)
            n95 = call <vilib>:"Add State(s) to Queue__jki_lib_state_machine.vi"("State(s) in Front (\"\")"="Instrument: Close\nData: Cleanup\nEvents: Unregister", "State(s) in (\"\")"="Process: Sync", "State(s) at Back (\"\")"="Exit") -> ("States Out"=w276:string)  [unwired: 12 in]
            n96 = call <vilib>:"Add State(s) to Queue__jki_lib_state_machine.vi"("State(s) in (\"\")"=w281, "State(s) at Back (\"\")"=w276) -> ("States Out"=w280:string)  [unwired: 13 in]
            n97 = call <vilib>:"Add State(s) to Queue__jki_lib_state_machine.vi"("State(s) in Front (\"\")"=w280, "State(s) in (\"\")"=w287) -> ("States Out"=w286:string)  [unwired: 13 in]
          }
          frame "---------- Process ----------" {
            # "Template Separator\n(You can make a copy of, or modify, this frame)"
            n98 = call <vilib>:"Add State(s) to Queue__jki_lib_state_machine.vi"("State(s) in (\"\")"=w292) -> ("States Out"=w291:string)  [unwired: 14 in]
          }
          frame "Process: Sync" {
            n99 = Unbundle By Name(w300) -> ("SMO"=w296:refnum<class "instrument.Cryostation.lvclass">)
            n100 = call <vilib>:"WaitOnProcessSync.vi"("error in (no error)"=w295, "SMO"=w296) -> ("error out"=w294:errorcluster, "Don't run?"=w299:bool)  [unwired: 7 in, 1 out]
            n101 = Select(t="Data: Cleanup\nEvents: Unregister\nExit", s=w299, f="") -> (s? t:f=w293:string)
            n102 = call <vilib>:"Add State(s) to Queue__jki_lib_state_machine.vi"("State(s) in Front (\"\")"=w293, "State(s) in (\"\")"=w303) -> ("States Out"=w302:string)  [unwired: 13 in]
          }
          frame "---------- Events ----------" {
            # "Template Separator\n(You can make a copy of, or modify, this frame)"
            n103 = call <vilib>:"Add State(s) to Queue__jki_lib_state_machine.vi"("State(s) in (\"\")"=w308) -> ("States Out"=w307:string)  [unwired: 14 in]
          }
          frame "Events: Register" {
            # "Expand to add\nmore events"
            n104 = Unbundle By Name(w316) -> ("SMO"=w313:refnum<class "instrument.Cryostation.lvclass">)
            n105 = call <vilib>:"GetProtectedEvents.vi"("SMO"=w313) -> ("error out"=w309:errorcluster, "SMO Protected Events"=w314:T6)  [unwired: 8 in, 1 out]
            n106 = register-events(w314) -> (reference out=w315:refnum<event-registration>, error out=w310:errorcluster)  [unwired: 2 in]
            n107 = Merge Errors(w312, w310, w309) -> (w311:errorcluster)
            n108 = call <vilib>:"Add State(s) to Queue__jki_lib_state_machine.vi"("State(s) in (\"\")"=w318) -> ("States Out"=w317:string)  [unwired: 14 in]
          }
          frame "Events: Unregister" {
            n109 = Unregister For Events(event registration refnum=w321, error in=w320) -> (error out=w319:errorcluster)
            n110 = call <vilib>:"Clear Errors.vi"("error in (no error)"=w319) -> ()  [unwired: 5 in, 2 out]
            n111 = call <vilib>:"Add State(s) to Queue__jki_lib_state_machine.vi"("State(s) in (\"\")"=w324) -> ("States Out"=w323:string)  [unwired: 14 in]
          }
          frame "---------- Instrument ----------" {
            # "Template Separator\n(You can make a copy of, or modify, this frame)"
            n112 = call <vilib>:"Add State(s) to Queue__jki_lib_state_machine.vi"("State(s) in (\"\")"=w329) -> ("States Out"=w328:string)  [unwired: 14 in]
          }
          frame "Instrument: Open" {
            n113 = Unbundle By Name(w332) -> ("SMO"=w335:refnum<class "instrument.Cryostation.lvclass">)
            n114 = call-dynamic "Open Hardware.vi"("error in (no error)"=w330, "instrument.Cryostation in"=w335) -> ("error out"=w331:errorcluster, "instrument.Cryostation out"=w334:refnum<class "instrument.Cryostation.lvclass">)  [unwired: 8 in]
            n115 = Bundle By Name(cluster=w332, "SMO"=w334) -> (w333:T3)
            n116 = call <vilib>:"Add State(s) to Queue__jki_lib_state_machine.vi"("State(s) in (\"\")"=w338) -> ("States Out"=w337:string)  [unwired: 14 in]
          }
          frame "Instrument: getAll" {
            n117 = Unbundle By Name(w345) -> ("SMO"=w347:refnum<class "instrument.Cryostation.lvclass">)
            n118 = call "Cryostation.getAll.vi"("error in (no error)"=w344, "instrument.Cryostation in"=w347) -> ("error out"=w340:errorcluster, "getAll"=w342:T7, "instrument.Cryostation out"=w343:refnum<class "instrument.Cryostation.lvclass">)  [unwired: 7 in]
            n119 = call <userlib>:"setAllData.vi"("error in (no error)"=w340, "AllData"=w342, "Instrument in"=w343) -> ("error out"=w339:errorcluster, "Instrument out"=w341:refnum<class "instrument.Cryostation.lvclass">)  [unwired: 7 in]
            n120 = Bundle By Name(cluster=w345, "SMO"=w341) -> (w346:T3)
            n121 = call <vilib>:"Add State(s) to Queue__jki_lib_state_machine.vi"("State(s) in (\"\")"=w350) -> ("States Out"=w349:string)  [unwired: 14 in]
          }
          frame "Instrument: Log" {
            n122 = Unbundle By Name(w359) -> ("SMO"=w355:refnum<class "instrument.Cryostation.lvclass">)
            n123 = Unbundle By Name(w355) -> ("getAll"=w351:T7)
            n124 = call-dynamic "Get SMO Database Paths.vi"("error in (no error)"=w354, "instrument.Cryostation in"=w355) -> ("error out"=w353:errorcluster, "Paths"=w358:string, "instrument.Cryostation out"=w357:refnum<class "instrument.Cryostation.lvclass">)  [unwired: 7 in]
            n125 = call <userlib>:"Instrument.logToDatabase.vi"("error in (no error)"=w353, "Data"=w351, "Paths"=w358, "Instrument"=w357) -> ("error out"=w352:errorcluster, "Instrument out"=w356:refnum<class "instrument.Cryostation.lvclass">)  [unwired: 6 in]
            n126 = Bundle By Name(cluster=w359, "SMO"=w356) -> (w360:T3)
            n127 = call <vilib>:"Add State(s) to Queue__jki_lib_state_machine.vi"("State(s) in (\"\")"=w363) -> ("States Out"=w362:string)  [unwired: 14 in]
          }
          frame "Instrument: Close" {
            n128 = Unbundle By Name(w366) -> ("SMO"=w369:refnum<class "instrument.Cryostation.lvclass">)
            n129 = call-dynamic "Close Hardware.vi"("error in (no error)"=w364, "instrument.Cryostation in"=w369) -> ("error out"=w365:errorcluster, "instrument.Cryostation out"=w368:refnum<class "instrument.Cryostation.lvclass">)  [unwired: 8 in]
            n130 = Bundle By Name(cluster=w366, "SMO"=w368) -> (w367:T3)
            n131 = call <vilib>:"Add State(s) to Queue__jki_lib_state_machine.vi"("State(s) in (\"\")"=w372) -> ("States Out"=w371:string)  [unwired: 14 in]
          }
        }
      }
    }
    frame Error {
    }
  }
  n132 = call-parent "Process.vi"("error in"=w5, "Instrument"=w4) -> ("error out"=w2:errorcluster, "Instrument out"=→"instrument.Cryostation out":refnum<class "instrument.Cryostation.lvclass">)  [unwired: 8 in]
  n133 = Merge Errors(w2, w1) -> (→"error out":errorcluster)
